vi "Write Temperature Task.vi"(8 "error in (no error)":errorcluster, 10 "Temperature Task":refnum<k21>, 11 "Humidifier in":refnum<class "Humidifier.lvclass">) -> (0 "error out":errorcluster, 3 "Humidifier out":refnum<class "Humidifier.lvclass">)   [LabVIEW 2014, in "Humidifier Lib.lvlib" / "Humidifier.lvclass"]
uses:
  Humidifier.lvclass
  Humidifier.lvclass/Humidifier.ctl
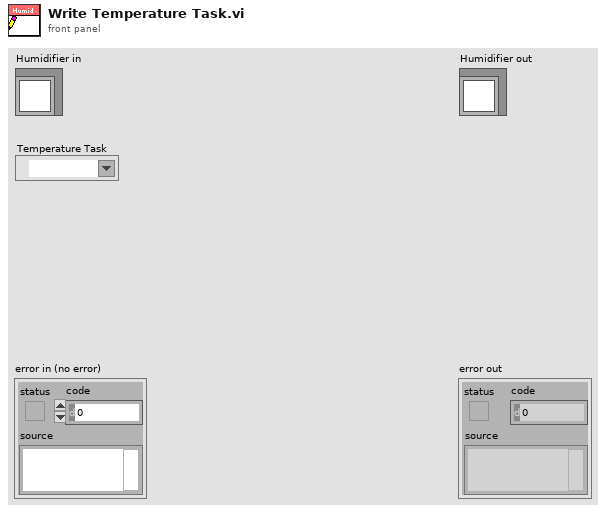
[diagram p1: front panel]
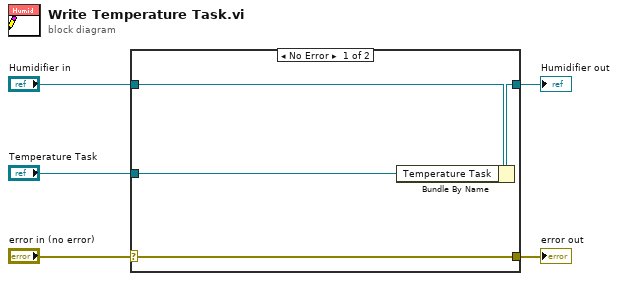
[diagram p0: block diagram]
diagram:
  n1 = case shown="No Error" "error in (no error)" {
    selector: "error in (no error)" -> [w9 w10]
    tunnel: [w9 w10] -> w4
    tunnel: [w7 w11] -> w2
    tunnel: "Humidifier in" -> [w8 w11]
    tunnel: "Temperature Task" -> [w6 _]
    frame No Error {
      n2 = Bundle By Name(cluster=w8, "Temperature Task"=w6) -> (w7:refnum<class "Humidifier.lvclass">)
    }
    frame Error {
    }
  }
  "error out" <- w4
  "Humidifier out" <- w2
